vi "Create All Message Queues.vi"(8 "error in (no error)":errorcluster caption="错误输入（无错误）") -> (0 "error out":errorcluster caption="错误输出", 3 "Message Queues out":T1 caption="消息队列输出")   [LabVIEW 2013, in "Message Queue.lvlib"]
doc: "本VI用于创建应用程序所需的所有消息队列。如应用程序需要两个以上消息队列，可右键单击上面的“消息队列”常量并选择“打开自定义类型”，将新的消息队列添加至该自定义类型，然后通过本VI进行初始化。"
uses:
  Message Queue.lvlib
  All Message Queues.ctl
  Message Cluster.ctl
  Enqueue Message (Single).vi
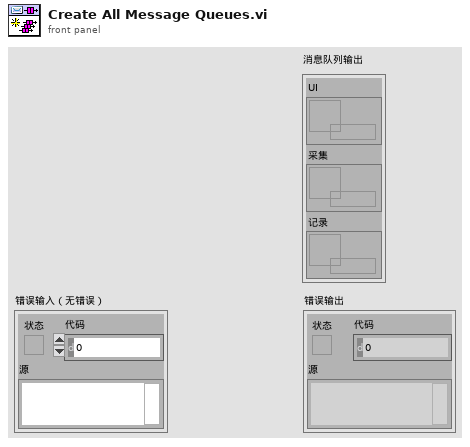
[diagram p1: front panel]
types:
  T1 = typedef "Message Queue.lvlib/All Message Queues.ctl" = cluster{"UI":refnum<queue>, "Acquisition":refnum<queue>, "Logging":refnum<queue>}
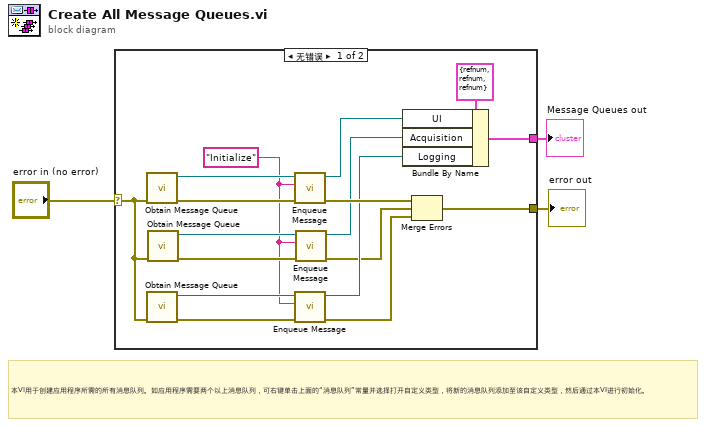
[diagram p0: block diagram]
diagram:
  # "本VI用于创建应用程序所需的所有消息队列。如应用程序需要两个以上消息队列，可右键单击上面的“消息队列”常量并选择打开自定义类型，将新的消息队列添加至该自定义类型，然后通过本VI进行初始化。"
  n1 = case shown="无错误" "error in (no error)" {
    selector: "error in (no error)" -> [w11 w21]
    tunnel: [w6 w21] -> w3
    tunnel: [w18 _] -> w2
    frame No Error {
      w10 = "Initialize" ("Message")
      n2 = call "Obtain Message Queue.vi"("error in (no error)"=w11) -> ("error out"=w17:errorcluster, "Message Queue"=w16:refnum<queue>)  [unwired: 9 in]
      n3 = call "Obtain Message Queue.vi"("error in (no error)"=w11) -> ("error out"=w13:errorcluster, "Message Queue"=w12:refnum<queue>)  [unwired: 9 in]
      n4 = call "Obtain Message Queue.vi"("error in (no error)"=w11) -> ("error out"=w14:errorcluster, "Message Queue"=w15:refnum<queue>)  [unwired: 9 in]
      n5 = call-poly "Enqueue Message.vi"("error in (no error)"=w17, "Message"=w10, "Message Queue"=w16) -> ("error out"=w20:errorcluster, "dup Message Queue"=w9:refnum<queue>)  [unwired: 7 in]
      n6 = call-poly "Enqueue Message.vi"("error in (no error)"=w13, "Message"=w10, "Message Queue"=w12) -> ("error out"=w4:errorcluster, "dup Message Queue"=w7:refnum<queue>)  [unwired: 7 in]
      n7 = call-poly "Enqueue Message.vi"("error in (no error)"=w14, "Message"=w10, "Message Queue"=w15) -> ("error out"=w5:errorcluster, "dup Message Queue"=w8:refnum<queue>)  [unwired: 7 in]
      n8 = Bundle By Name(cluster=T1 {"UI"=refnum, "Acquisition"=refnum, "Logging"=refnum} ("Message Queues"), "UI"=w9, "Acquisition"=w8, "Logging"=w7) -> (w18:T1)
      n9 = Merge Errors(w20, w5, w4) -> (w6:errorcluster)
    }
    frame Error {
    }
  }
  "Message Queues out" <- w2
  "error out" <- w3
